vi "picoharp_structmaker3.vi"(0 "Channel 3 Zero Cross":i32, 1 "Channel 2 Zero Cross":i32, 2 "Channel 1 Zero Cross":i32, 3 "Channel 0 Zero Cross":i32, 4 "Channel 3 Discriminator":i32, 5 "Channel 2 Discriminator":i32, 6 "Channel 1 Discriminator":i32, 7 "Channel 0 Discriminator":i32, 8 "n_records":i32=1597208, 9 "Use user inputs?":bool, 11 "Measurement Mode":i32(ring) items=["Interactive", "Reserved", "T2", "T3"], 13 "Binning":i32(ring) items=["Base", "x2", "x4", "x8", "x16", "x32", "x64", "x128", "x256", "x512", "x1024"], 15 "COMMENT":string, 17 "Acquisition Time":i32, 19 "Stop after (ms)":i32, 20 "Sync Offset":i32, 21 "Sync input Zero Cross Level":i32, 22 "Sync input Discriminator (mv)":i32, 23 "Sync Divider":i32(ring) items=["0", "2", "4", "8"], 24 "Channel 3 Offset":i32, 25 "Channel  2 Offset":i32, 26 "Channel 1 offset":i32, 27 "Channel 0 offset":i32) -> (12 "Resolution":dbl, 14 "Header in binary":u8[](array[numeric]), 18 "Cluster":T1)   [LabVIEW 2015, in "picoharp.lvclass"]
uses:
  picoharp.lvclass
panel:
  in  "?":bool
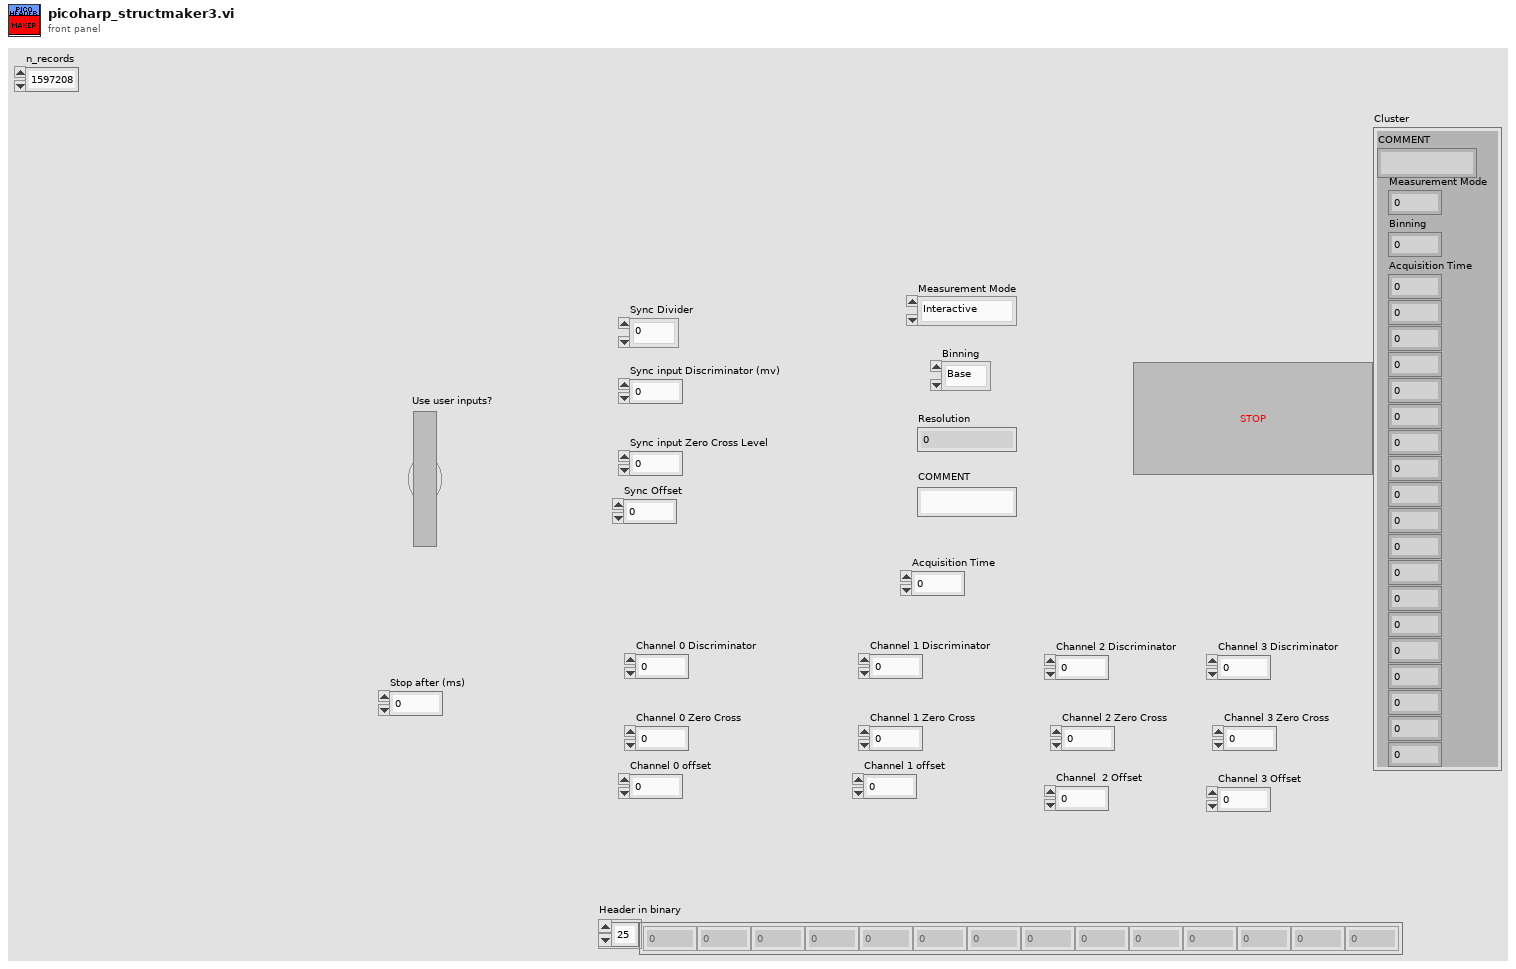
[diagram p1: front panel]
types:
  T1 = cluster{"COMMENT":string, "Measurement Mode":i32, "Binning":i32, "Acquisition Time":i32, i32, i32, i32, i32, i32, i32, i32, i32, i32, i32, i32, i32, i32, i32, i32, i32, i32, i64}
  T2 = cluster{"COMMENT 2":string, "Measurement Mode 2":i32, "Binning 2":i32, "Acquisition Time 2":i32, i32, i32, i32, i32, i32, i32, i32, i32, i32, i32, i32, i32, i32, i32, i32, i32, i32, i64}
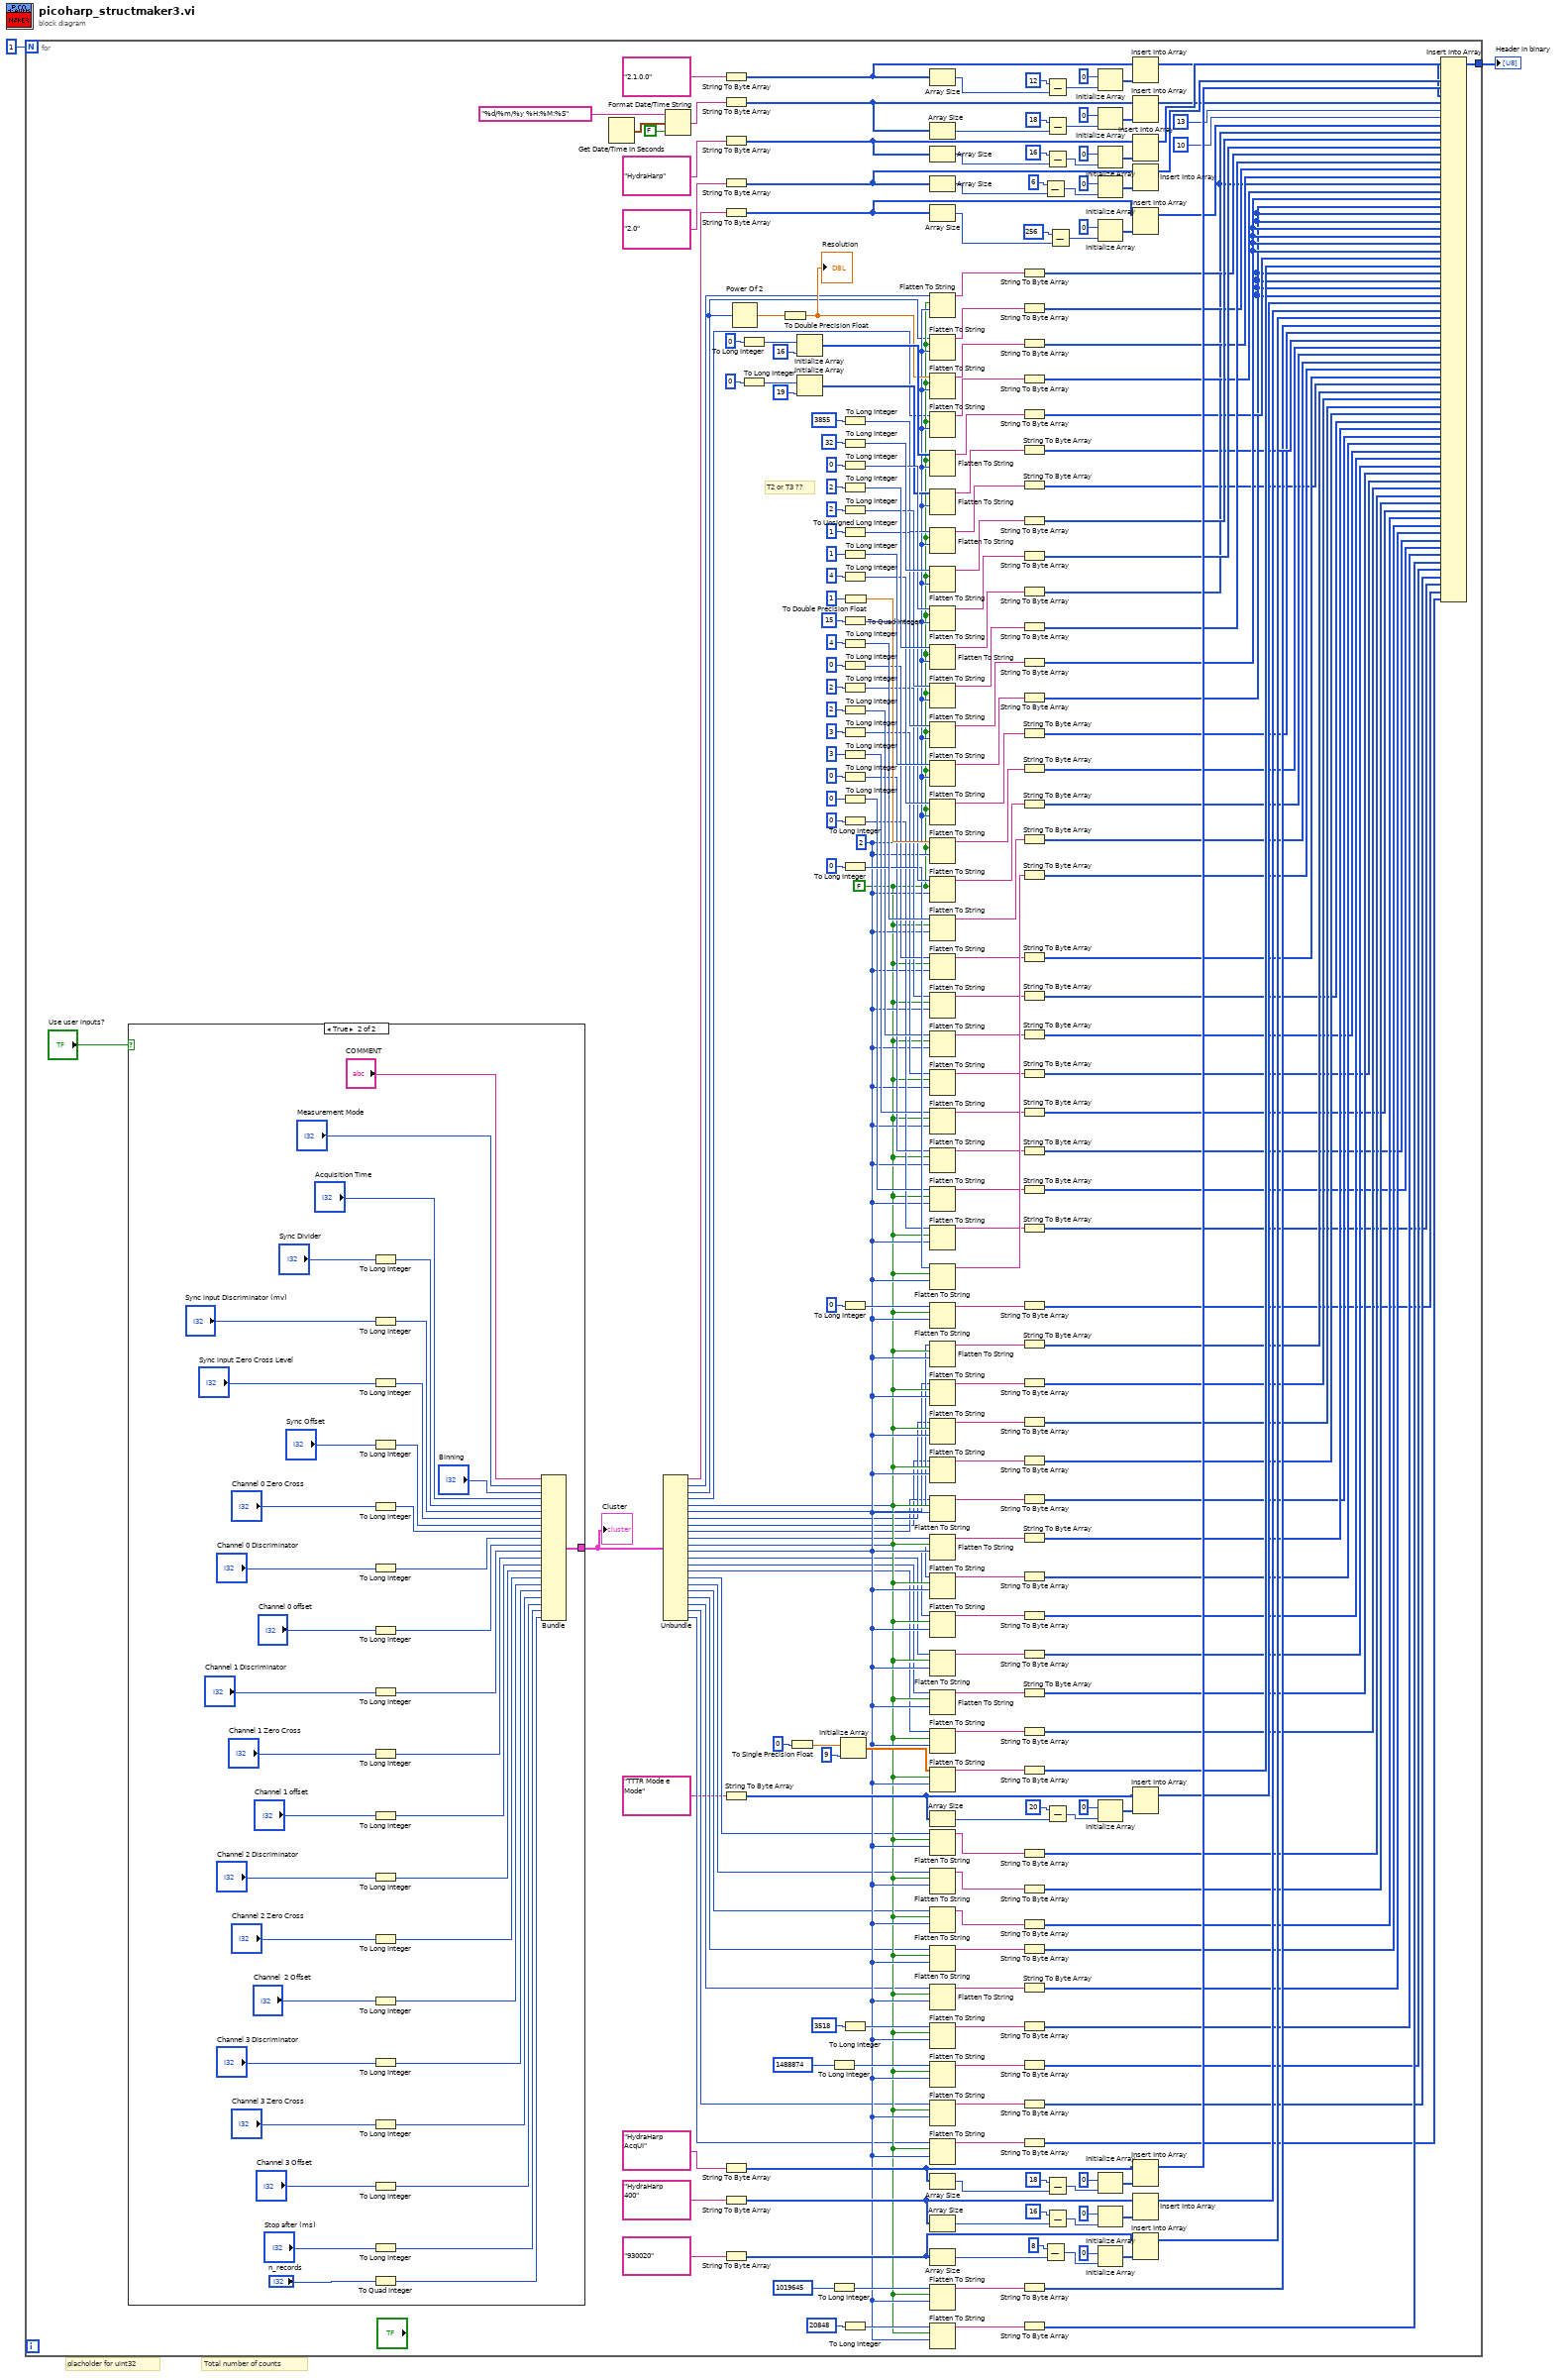
[diagram p0: block diagram]
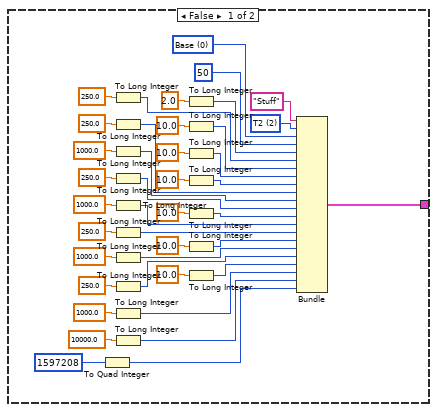
[diagram p2: hidden frame]
diagram:
  # "Total number of counts"
  # "placholder for uint32"
  n1 = for {
    N: 1 -> [_]
    tunnel: [w261] -> w2
    w31 = 2
    w30 = FALSE
    # "T2 or T3 ??"
    n2 = case shown="True" "Use user inputs?" {
      tunnel: [w270 w332] -> w3
      frame False {
        w292 = 2 items=["Interactive", "Reserved", "T2", "T3"] ("Measurement Mode 2")
        w291 = 0 items=["Base", "x2", "x4", "x8", "x16", "x32", "x64", "x128", "x256", "x512", "x1024"] ("Binning 2")
        n3 = To Quad Integer(1:1597208) -> (0:w271:i64)
        n4 = To Long Integer(number=250.0 ("Sync input Discriminator (mv) 2")) -> (32bit integer=w288:i32)
        n5 = To Long Integer(number=250.0 ("Channel 0 Discriminator 2")) -> (32bit integer=w281:i32)
        n6 = To Long Integer(number=1000.0 ("Channel 0 offset 2")) -> (32bit integer=w285:i32)
        n7 = To Long Integer(number=250.0 ("Channel 1 Discriminator  2")) -> (32bit integer=w284:i32)
        n8 = To Long Integer(number=1000.0 ("Channel 1 offset  2")) -> (32bit integer=w280:i32)
        n9 = To Long Integer(number=250.0 ("Channel 2 Discriminator 2")) -> (32bit integer=w279:i32)
        n10 = To Long Integer(number=1000.0 ("Channel  2 Offset 2")) -> (32bit integer=w277:i32)
        n11 = To Long Integer(number=250.0 ("Channel 3 Discriminator 2")) -> (32bit integer=w276:i32)
        n12 = To Long Integer(number=1000.0 ("Channel 3 Offset 2")) -> (32bit integer=w274:i32)
        n13 = To Long Integer(number=10000.0 ("Stop after (ms) 2")) -> (32bit integer=w273:i32)
        n14 = To Long Integer(number=2.0 ("Sync Divider 2")) -> (32bit integer=w289:i32)
        n15 = To Long Integer(number=10.0 ("Sync input Zero Cross Level 2")) -> (32bit integer=w287:i32)
        n16 = To Long Integer(number=10.0 ("Sync Offset 2")) -> (32bit integer=w282:i32)
        n17 = To Long Integer(number=10.0 ("Channel 0 Zero Cross 2")) -> (32bit integer=w286:i32)
        n18 = To Long Integer(number=10.0 ("Channel 1 Zero Cross  2")) -> (32bit integer=w283:i32)
        n19 = To Long Integer(number=10.0 ("Channel 2 Zero Cross 2")) -> (32bit integer=w278:i32)
        n20 = To Long Integer(number=10.0 ("Channel 3 Zero Cross 2")) -> (32bit integer=w275:i32)
        n21 = Bundle("COMMENT 2"="Stuff", "Measurement Mode 2"=w292, "Binning 2"=w291, "Acquisition Time 2"=50, w289, w288, w287, w282, w286, w281, w285, w284, w283, w280, w279, w278, w277, w276, w275, w274, w273, w271) -> (w270:T2)  [unwired: 1 in]
      }
      frame True {
        n22 = To Long Integer(number="Sync Divider") -> (32bit integer=w328:i32)
        n23 = To Long Integer(number="Sync input Discriminator (mv)") -> (32bit integer=w327:i32)
        n24 = To Long Integer(number="Sync input Zero Cross Level") -> (32bit integer=w326:i32)
        n25 = To Long Integer(number="Sync Offset") -> (32bit integer=w321:i32)
        n26 = To Long Integer(number="Channel 0 Zero Cross") -> (32bit integer=w325:i32)
        n27 = To Long Integer(number="Channel 0 Discriminator") -> (32bit integer=w320:i32)
        n28 = To Long Integer(number="Channel 0 offset") -> (32bit integer=w324:i32)
        n29 = To Long Integer(number="Channel 1 Discriminator") -> (32bit integer=w323:i32)
        n30 = To Long Integer(number="Channel 1 Zero Cross") -> (32bit integer=w322:i32)
        n31 = To Long Integer(number="Channel 1 offset") -> (32bit integer=w319:i32)
        n32 = To Long Integer(number="Channel 2 Discriminator") -> (32bit integer=w318:i32)
        n33 = To Long Integer(number="Channel 2 Zero Cross") -> (32bit integer=w317:i32)
        n34 = To Long Integer(number="Channel  2 Offset") -> (32bit integer=w316:i32)
        n35 = To Long Integer(number="Channel 3 Discriminator") -> (32bit integer=w315:i32)
        n36 = To Long Integer(number="Channel 3 Zero Cross") -> (32bit integer=w314:i32)
        n37 = To Long Integer(number="Channel 3 Offset") -> (32bit integer=w313:i32)
        n38 = To Long Integer(number="Stop after (ms)") -> (32bit integer=w312:i32)
        n39 = To Quad Integer(1:"n_records") -> (0:w311:i64)
        n40 = Bundle("COMMENT"="COMMENT", "Measurement Mode"="Measurement Mode", "Binning"="Binning", "Acquisition Time"="Acquisition Time", w328, w327, w326, w321, w325, w320, w324, w323, w322, w319, w318, w317, w316, w315, w314, w313, w312, w311) -> (w332:T1)  [unwired: 1 in]
      }
    }
    "Cluster" <- w3
    n41 = Get Date/Time In Seconds() -> (seconds since 1Jan1904=w229:timestamp)
    n42 = Unbundle(w3) -> ("COMMENT"=w27:string, "Measurement Mode"=w26:i32, "Binning"=w25:i32, "Acquisition Time"=w24:i32, w23:i32, w22:i32, w21:i32, w19:i32, w20:i32, w15:i32, w16:i32, w17:i32, w18:i32, w14:i32, w13:i32, w12:i32, w11:i32, w10:i32, w9:i32, w8:i32, w7:i32, w6:i64)
    n43 = Format Date/Time String(time format string (%c)="%d/%m/%y %H:%M:%S", seconds (now)=w229, UTC format=FALSE) -> (date/time string=w227:string)
    n44 = String To Byte Array(string="2.1.0.0") -> (unsigned byte array=w231:u8[])
    n45 = String To Byte Array(string=w227) -> (unsigned byte array=w230:u8[])
    n46 = String To Byte Array(string="HydraHarp") -> (unsigned byte array=w256:u8[])
    n47 = String To Byte Array(string="2.0") -> (unsigned byte array=w260:u8[])
    n48 = String To Byte Array(string=w27) -> (unsigned byte array=w218:u8[])
    n49 = String To Byte Array(string="TTTR Mode e Mode") -> (unsigned byte array=w168:u8[])
    n50 = String To Byte Array(string="HydraHarp AcqUI") -> (unsigned byte array=w245:u8[])
    n51 = String To Byte Array(string="HydraHarp 400") -> (unsigned byte array=w160:u8[])
    n52 = String To Byte Array(string="930020") -> (unsigned byte array=w152:u8[])
    n53 = Power Of 2(x=w25) -> (2^x=w131:dbl)
    n54 = To Long Integer(number=0) -> (32bit integer=w183:i32)
    n55 = To Long Integer(number=0) -> (32bit integer=w147:i32)
    n56 = To Double Precision Float(number=w131) -> (double precision float=w130:dbl)
    "Resolution" <- w130
    n57 = To Single Precision Float(number=0) -> (single precision float=w175:sgl)
    n58 = Initialize Array(w183, 16) -> (w182:i32[])
    n59 = Initialize Array(w147, 19) -> (w146:i32[])
    n60 = To Long Integer(number=1488874) -> (32bit integer=w43:i32)
    n61 = To Long Integer(number=1019645) -> (32bit integer=w142:i32)
    n62 = Initialize Array(w175, 9) -> (w174:sgl[])
    n63 = To Long Integer(number=3855) -> (32bit integer=w112:i32)
    n64 = To Long Integer(number=32) -> (32bit integer=w209:i32)
    n65 = To Long Integer(number=0) -> (32bit integer=w206:i32)
    n66 = To Long Integer(number=2) -> (32bit integer=w210:i32)
    n67 = To Long Integer(number=2) -> (32bit integer=w201:i32)
    n68 = To Unsigned Long Integer(number=1) -> (unsigned 32bit integer=w191:u32)
    n69 = To Long Integer(number=1) -> (32bit integer=w187:i32)
    n70 = To Long Integer(number=4) -> (32bit integer=w138:i32)
    n71 = To Quad Integer(1:15) -> (0:w127:i64)
    n72 = To Long Integer(number=4) -> (32bit integer=w122:i32)
    n73 = To Long Integer(number=0) -> (32bit integer=w115:i32)
    n74 = To Long Integer(number=2) -> (32bit integer=w101:i32)
    n75 = To Long Integer(number=2) -> (32bit integer=w91:i32)
    n76 = To Long Integer(number=3) -> (32bit integer=w76:i32)
    n77 = To Long Integer(number=3) -> (32bit integer=w66:i32)
    n78 = To Long Integer(number=0) -> (32bit integer=w57:i32)
    n79 = To Long Integer(number=0) -> (32bit integer=w52:i32)
    n80 = To Long Integer(number=0) -> (32bit integer=w36:i32)
    n81 = To Long Integer(number=0) -> (32bit integer=w119:i32)
    n82 = To Long Integer(number=0) -> (32bit integer=w34:i32)
    n83 = To Long Integer(number=3518) -> (32bit integer=w51:i32)
    n84 = To Long Integer(number=20848) -> (32bit integer=w50:i32)
    n85 = To Double Precision Float(number=1) -> (double precision float=w134:dbl)
    n86 = Array Size(array=w231) -> (size(s)=w243:i32)
    n87 = Array Size(array=w230) -> (size(s)=w240:i32)
    n88 = Array Size(array=w256) -> (size(s)=w254:i32)
    n89 = Array Size(array=w260) -> (size(s)=w258:i32)
    n90 = Array Size(array=w218) -> (size(s)=w223:i32)
    n91 = Flatten To String(anything=w26, prepend array or string size? (T)=w30, byte order (0:big-endian, network order)=w31) -> (data string=w205:string)  [unwired: 1 in, 2 out]
    n92 = Flatten To String(anything=w25, prepend array or string size? (T)=w30, byte order (0:big-endian, network order)=w31) -> (data string=w199:string)  [unwired: 1 in, 2 out]
    n93 = Flatten To String(anything=w130, prepend array or string size? (T)=w30, byte order (0:big-endian, network order)=w31) -> (data string=w197:string)  [unwired: 1 in, 2 out]
    n94 = Flatten To String(anything=w24, prepend array or string size? (T)=w30, byte order (0:big-endian, network order)=w31) -> (data string=w195:string)  [unwired: 1 in, 2 out]
    n95 = Flatten To String(anything=w182, prepend array or string size? (T)=w30, byte order (0:big-endian, network order)=w31) -> (data string=w181:string)  [unwired: 1 in, 2 out]
    n96 = Flatten To String(anything=w146, byte order (0:big-endian, network order)=w31) -> (data string=w145:string)  [unwired: 2 in, 2 out]
    n97 = Flatten To String(anything=w112, prepend array or string size? (T)=w30, byte order (0:big-endian, network order)=w31) -> (data string=w114:string)  [unwired: 1 in, 2 out]
    n98 = Flatten To String(anything=w209, prepend array or string size? (T)=w30, byte order (0:big-endian, network order)=w31) -> (data string=w215:string)  [unwired: 1 in, 2 out]
    n99 = Flatten To String(anything=w206, prepend array or string size? (T)=w30, byte order (0:big-endian, network order)=w31) -> (data string=w213:string)  [unwired: 1 in, 2 out]
    n100 = Flatten To String(anything=w210, prepend array or string size? (T)=w30, byte order (0:big-endian, network order)=w31) -> (data string=w216:string)  [unwired: 1 in, 2 out]
    n101 = Flatten To String(anything=w201, prepend array or string size? (T)=w30, byte order (0:big-endian, network order)=w31) -> (data string=w203:string)  [unwired: 1 in, 2 out]
    n102 = Flatten To String(anything=w191, prepend array or string size? (T)=w30, byte order (0:big-endian, network order)=w31) -> (data string=w192:string)  [unwired: 1 in, 2 out]
    n103 = Flatten To String(anything=w187, prepend array or string size? (T)=w30, byte order (0:big-endian, network order)=w31) -> (data string=w189:string)  [unwired: 1 in, 2 out]
    n104 = Flatten To String(anything=w138, prepend array or string size? (T)=w30, byte order (0:big-endian, network order)=w31) -> (data string=w137:string)  [unwired: 1 in, 2 out]
    n105 = Flatten To String(anything=w134, prepend array or string size? (T)=w30, byte order (0:big-endian, network order)=w31) -> (data string=w133:string)  [unwired: 1 in, 2 out]
    n106 = Flatten To String(anything=w127, prepend array or string size? (T)=w30, byte order (0:big-endian, network order)=w31) -> (data string=w129:string)  [unwired: 1 in, 2 out]
    n107 = Flatten To String(anything=w122, prepend array or string size? (T)=w30, byte order (0:big-endian, network order)=w31) -> (data string=w126:string)  [unwired: 1 in, 2 out]
    n108 = Flatten To String(anything=w115, prepend array or string size? (T)=w30, byte order (0:big-endian, network order)=w31) -> (data string=w117:string)  [unwired: 1 in, 2 out]
    n109 = Flatten To String(anything=w101, prepend array or string size? (T)=w30, byte order (0:big-endian, network order)=w31) -> (data string=w100:string)  [unwired: 1 in, 2 out]
    n110 = Flatten To String(anything=w91, prepend array or string size? (T)=w30, byte order (0:big-endian, network order)=w31) -> (data string=w90:string)  [unwired: 1 in, 2 out]
    n111 = Flatten To String(anything=w76, prepend array or string size? (T)=w30, byte order (0:big-endian, network order)=w31) -> (data string=w80:string)  [unwired: 1 in, 2 out]
    n112 = Flatten To String(anything=w66, prepend array or string size? (T)=w30, byte order (0:big-endian, network order)=w31) -> (data string=w70:string)  [unwired: 1 in, 2 out]
    n113 = Flatten To String(anything=w57, prepend array or string size? (T)=w30, byte order (0:big-endian, network order)=w31) -> (data string=w56:string)  [unwired: 1 in, 2 out]
    n114 = Flatten To String(anything=w52, prepend array or string size? (T)=w30, byte order (0:big-endian, network order)=w31) -> (data string=w55:string)  [unwired: 1 in, 2 out]
    n115 = Flatten To String(anything=w36, prepend array or string size? (T)=w30, byte order (0:big-endian, network order)=w31) -> (data string=w37:string)  [unwired: 1 in, 2 out]
    n116 = Flatten To String(anything=w119, prepend array or string size? (T)=w30, byte order (0:big-endian, network order)=w31) -> (data string=w121:string)  [unwired: 1 in, 2 out]
    n117 = Flatten To String(anything=w34, prepend array or string size? (T)=w30, byte order (0:big-endian, network order)=w31) -> (data string=w35:string)  [unwired: 1 in, 2 out]
    n118 = Flatten To String(anything=w23, prepend array or string size? (T)=w30, byte order (0:big-endian, network order)=w31) -> (data string=w109:string)  [unwired: 1 in, 2 out]
    n119 = Flatten To String(anything=w22, prepend array or string size? (T)=w30, byte order (0:big-endian, network order)=w31) -> (data string=w108:string)  [unwired: 1 in, 2 out]
    n120 = Flatten To String(anything=w21, prepend array or string size? (T)=w30, byte order (0:big-endian, network order)=w31) -> (data string=w107:string)  [unwired: 1 in, 2 out]
    n121 = Flatten To String(anything=w19, prepend array or string size? (T)=w30, byte order (0:big-endian, network order)=w31) -> (data string=w106:string)  [unwired: 1 in, 2 out]
    n122 = Flatten To String(anything=w20, prepend array or string size? (T)=w30, byte order (0:big-endian, network order)=w31) -> (data string=w98:string)  [unwired: 1 in, 2 out]
    n123 = Flatten To String(anything=w15, prepend array or string size? (T)=w30, byte order (0:big-endian, network order)=w31) -> (data string=w99:string)  [unwired: 1 in, 2 out]
    n124 = Flatten To String(anything=w16, prepend array or string size? (T)=w30, byte order (0:big-endian, network order)=w31) -> (data string=w97:string)  [unwired: 1 in, 2 out]
    n125 = Flatten To String(anything=w17, prepend array or string size? (T)=w30, byte order (0:big-endian, network order)=w31) -> (data string=w87:string)  [unwired: 1 in, 2 out]
    n126 = Flatten To String(anything=w18, prepend array or string size? (T)=w30, byte order (0:big-endian, network order)=w31) -> (data string=w88:string)  [unwired: 1 in, 2 out]
    n127 = Flatten To String(anything=w14, prepend array or string size? (T)=w30, byte order (0:big-endian, network order)=w31) -> (data string=w89:string)  [unwired: 1 in, 2 out]
    n128 = Flatten To String(anything=w13, prepend array or string size? (T)=w30, byte order (0:big-endian, network order)=w31) -> (data string=w77:string)  [unwired: 1 in, 2 out]
    n129 = Flatten To String(anything=w174, prepend array or string size? (T)=w30, byte order (0:big-endian, network order)=w31) -> (data string=w178:string)  [unwired: 1 in, 2 out]
    n130 = Array Size(array=w168) -> (size(s)=w172:i32)
    n131 = Flatten To String(anything=w12, prepend array or string size? (T)=w30, byte order (0:big-endian, network order)=w31) -> (data string=w78:string)  [unwired: 1 in, 2 out]
    n132 = Flatten To String(anything=w11, prepend array or string size? (T)=w30, byte order (0:big-endian, network order)=w31) -> (data string=w79:string)  [unwired: 1 in, 2 out]
    n133 = Flatten To String(anything=w10, prepend array or string size? (T)=w30, byte order (0:big-endian, network order)=w31) -> (data string=w67:string)  [unwired: 1 in, 2 out]
    n134 = Flatten To String(anything=w9, prepend array or string size? (T)=w30, byte order (0:big-endian, network order)=w31) -> (data string=w68:string)  [unwired: 1 in, 2 out]
    n135 = Flatten To String(anything=w8, prepend array or string size? (T)=w30, byte order (0:big-endian, network order)=w31) -> (data string=w69:string)  [unwired: 1 in, 2 out]
    n136 = Flatten To String(anything=w51, prepend array or string size? (T)=w30, byte order (0:big-endian, network order)=w31) -> (data string=w54:string)  [unwired: 1 in, 2 out]
    n137 = Flatten To String(anything=w43, prepend array or string size? (T)=w30, byte order (0:big-endian, network order)=w31) -> (data string=w45:string)  [unwired: 1 in, 2 out]
    n138 = Flatten To String(anything=w7, prepend array or string size? (T)=w30, byte order (0:big-endian, network order)=w31) -> (data string=w41:string)  [unwired: 1 in, 2 out]
    n139 = Flatten To String(anything=w6, prepend array or string size? (T)=w30, byte order (0:big-endian, network order)=w31) -> (data string=w29:string)  [unwired: 1 in, 2 out]
    n140 = Array Size(array=w245) -> (size(s)=w250:i32)
    n141 = Array Size(array=w160) -> (size(s)=w164:i32)
    n142 = Array Size(array=w152) -> (size(s)=w156:i32)
    n143 = Flatten To String(anything=w142, prepend array or string size? (T)=w30, byte order (0:big-endian, network order)=w31) -> (data string=w141:string)  [unwired: 1 in, 2 out]
    n144 = Flatten To String(anything=w50, prepend array or string size? (T)=w30, byte order (0:big-endian, network order)=w31) -> (data string=w53:string)  [unwired: 1 in, 2 out]
    n145 = String To Byte Array(string=w205) -> (unsigned byte array=w204:u8[])
    n146 = String To Byte Array(string=w199) -> (unsigned byte array=w198:u8[])
    n147 = String To Byte Array(string=w197) -> (unsigned byte array=w196:u8[])
    n148 = String To Byte Array(string=w195) -> (unsigned byte array=w194:u8[])
    n149 = String To Byte Array(string=w181) -> (unsigned byte array=w180:u8[])
    n150 = String To Byte Array(string=w145) -> (unsigned byte array=w144:u8[])
    n151 = String To Byte Array(string=w114) -> (unsigned byte array=w110:u8[])
    n152 = String To Byte Array(string=w215) -> (unsigned byte array=w214:u8[])
    n153 = String To Byte Array(string=w213) -> (unsigned byte array=w212:u8[])
    n154 = String To Byte Array(string=w216) -> (unsigned byte array=w193:u8[])
    n155 = String To Byte Array(string=w203) -> (unsigned byte array=w200:u8[])
    n156 = String To Byte Array(string=w192) -> (unsigned byte array=w186:u8[])
    n157 = String To Byte Array(string=w189) -> (unsigned byte array=w150:u8[])
    n158 = String To Byte Array(string=w137) -> (unsigned byte array=w136:u8[])
    n159 = String To Byte Array(string=w133) -> (unsigned byte array=w132:u8[])
    n160 = String To Byte Array(string=w129) -> (unsigned byte array=w125:u8[])
    n161 = String To Byte Array(string=w126) -> (unsigned byte array=w124:u8[])
    n162 = String To Byte Array(string=w121) -> (unsigned byte array=w118:u8[])
    n163 = String To Byte Array(string=w117) -> (unsigned byte array=w111:u8[])
    n164 = String To Byte Array(string=w100) -> (unsigned byte array=w95:u8[])
    n165 = String To Byte Array(string=w90) -> (unsigned byte array=w85:u8[])
    n166 = String To Byte Array(string=w80) -> (unsigned byte array=w75:u8[])
    n167 = String To Byte Array(string=w70) -> (unsigned byte array=w65:u8[])
    n168 = String To Byte Array(string=w56) -> (unsigned byte array=w49:u8[])
    n169 = String To Byte Array(string=w55) -> (unsigned byte array=w48:u8[])
    n170 = String To Byte Array(string=w37) -> (unsigned byte array=w33:u8[])
    n171 = String To Byte Array(string=w35) -> (unsigned byte array=w32:u8[])
    n172 = String To Byte Array(string=w109) -> (unsigned byte array=w105:u8[])
    n173 = String To Byte Array(string=w108) -> (unsigned byte array=w104:u8[])
    n174 = String To Byte Array(string=w107) -> (unsigned byte array=w103:u8[])
    n175 = String To Byte Array(string=w106) -> (unsigned byte array=w102:u8[])
    n176 = String To Byte Array(string=w98) -> (unsigned byte array=w93:u8[])
    n177 = String To Byte Array(string=w99) -> (unsigned byte array=w94:u8[])
    n178 = String To Byte Array(string=w97) -> (unsigned byte array=w92:u8[])
    n179 = String To Byte Array(string=w87) -> (unsigned byte array=w84:u8[])
    n180 = String To Byte Array(string=w88) -> (unsigned byte array=w83:u8[])
    n181 = String To Byte Array(string=w89) -> (unsigned byte array=w82:u8[])
    n182 = String To Byte Array(string=w77) -> (unsigned byte array=w74:u8[])
    n183 = String To Byte Array(string=w178) -> (unsigned byte array=w177:u8[])
    n184 = String To Byte Array(string=w78) -> (unsigned byte array=w73:u8[])
    n185 = String To Byte Array(string=w79) -> (unsigned byte array=w72:u8[])
    n186 = String To Byte Array(string=w67) -> (unsigned byte array=w64:u8[])
    n187 = String To Byte Array(string=w68) -> (unsigned byte array=w63:u8[])
    n188 = String To Byte Array(string=w69) -> (unsigned byte array=w62:u8[])
    n189 = String To Byte Array(string=w54) -> (unsigned byte array=w47:u8[])
    n190 = String To Byte Array(string=w45) -> (unsigned byte array=w42:u8[])
    n191 = String To Byte Array(string=w41) -> (unsigned byte array=w40:u8[])
    n192 = String To Byte Array(string=w29) -> (unsigned byte array=w28:u8[])
    n193 = String To Byte Array(string=w141) -> (unsigned byte array=w140:u8[])
    n194 = String To Byte Array(string=w53) -> (unsigned byte array=w46:u8[])
    n195 = Subtract(x=6, y=w258) -> (x-y=w257:i32)
    n196 = Subtract(x=8, y=w156) -> (x-y=w154:i32)
    n197 = Subtract(x=12, y=w243) -> (x-y=w241:i32)
    n198 = Subtract(x=18, y=w240) -> (x-y=w238:i32)
    n199 = Subtract(x=16, y=w254) -> (x-y=w253:i32)
    n200 = Subtract(x=20, y=w172) -> (x-y=w170:i32)
    n201 = Subtract(x=18, y=w250) -> (x-y=w247:i32)
    n202 = Subtract(x=16, y=w164) -> (x-y=w162:i32)
    n203 = Subtract(x=256, y=w223) -> (x-y=w221:i32)
    n204 = Initialize Array(0, w241) -> (w232:i32[])
    n205 = Initialize Array(0, w238) -> (w233:i32[])
    n206 = Initialize Array(0, w253) -> (w268:i32[])
    n207 = Initialize Array(0, w257) -> (w266:i32[])
    n208 = Initialize Array(0, w221) -> (w219:i32[])
    n209 = Initialize Array(0, w170) -> (w169:i32[])
    n210 = Initialize Array(0, w247) -> (w249:i32[])
    n211 = Initialize Array(0, w162) -> (w161:i32[])
    n212 = Initialize Array(0, w154) -> (w153:i32[])
    n213 = Insert Into Array(array=w231, new element=w232) -> (w237:u8[])  [unwired: 1 in]
    n214 = Insert Into Array(array=w230, new element=w233) -> (w236:u8[])  [unwired: 1 in]
    n215 = Insert Into Array(array=w256, new element=w268) -> (w263:u8[])  [unwired: 1 in]
    n216 = Insert Into Array(array=w260, new element=w266) -> (w262:u8[])  [unwired: 1 in]
    n217 = Insert Into Array(array=w218, new element=w219) -> (w217:u8[])  [unwired: 1 in]
    n218 = Insert Into Array(array=w168, new element=w169) -> (w167:u8[])  [unwired: 1 in]
    n219 = Insert Into Array(array=w245, new element=w249) -> (w246:u8[])  [unwired: 1 in]
    n220 = Insert Into Array(array=w160, new element=w161) -> (w159:u8[])  [unwired: 1 in]
    n221 = Insert Into Array(array=w152, new element=w153) -> (w151:u8[])  [unwired: 1 in]
    n222 = Insert Into Array(array=w263, new element #1=w262, new element #2=w246, new element #3=w237, new element #4=w236, new element #5=u8 13, new element #6=u8 10, new element #7=w217, new element #8=w193, new element #9=w214, new element #10=w212, new element #11=w204, new element #12=w200, new element #13=w198, new element #14=w196, new element #15=w193, new element #16=w194, new element #17=w186, new element #18=w150, new element #19=w150, new element #20=w150, new element #21=w186, new element #22=w186, new element #23=w186, new element #24=w186, new element #25=w180, new element #26=w177, new element #27=w150, new element #28=w150, new element #29=w150, new element #30=w150, new element #31=w167, new element #32=w159, new element #33=w151, new element #34=w140, new element #35=w136, new element #36=w144, new element #37=w132, new element #38=w125, new element #39=w124, new element #40=w118, new element #41=w111, new element #42=w110, new element #43=w105, new element #44=w104, new element #45=w103, new element #46=w102, new element #47=w95, new element #48=w94, new element #49=w93, new element #50=w92, new element #51=w85, new element #52=w84, new element #53=w83, new element #54=w82, new element #55=w75, new element #56=w74, new element #57=w73, new element #58=w72, new element #59=w65, new element #60=w64, new element #61=w63, new element #62=w62, new element #63=w49, new element #64=w48, new element #65=w47, new element #66=w46, new element #67=w42, new element #68=w40, new element #69=w33, new element #70=w32, new element #71=w28) -> (w261:u8[])  [unwired: 1 in]
  }
  "Header in binary" <- w2
